vi "获取2号下位机4路温度值并显示和存进数据库.vi"() -> ()   [LabVIEW 2022 SP3]
uses:
  <vilib>/Instr/_visa.llb/VISA Configure Serial Port (Instr).vi
panel:
  out "所有测量记录":string[][](table)
  out "提取的第四路温度原始数据":string
  out "提取的第三路温度原始数据":string
  out "提取的第二路温度原始数据":string
  out "第一路温度值":dbl[](array[numeric])
  out "提取的第一路温度原始数据":string
  out "获取下位机返回的原始数据包":string
  in  "发送命令":string
  in  "波特率":u32=9600 caption="波特率(9600)"
  in  "选择串口":refnum<visa-resource-name>
  # "第二路温度值"
  # "第三路温度值"
  # "第四路温度值"
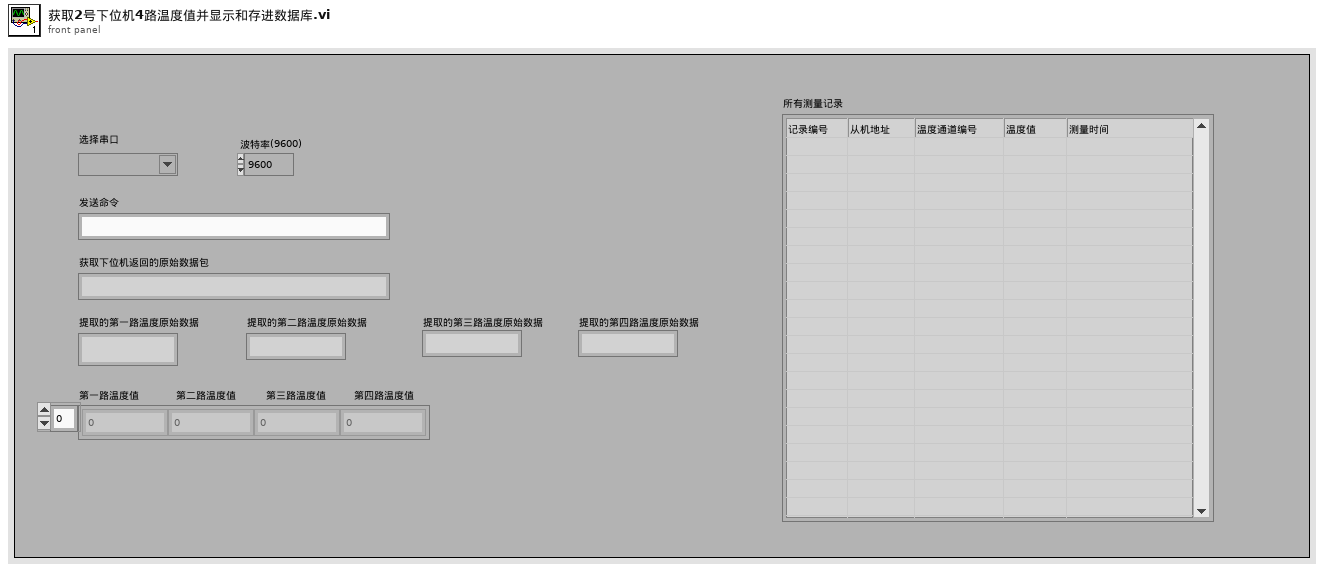
[diagram p1: front panel]
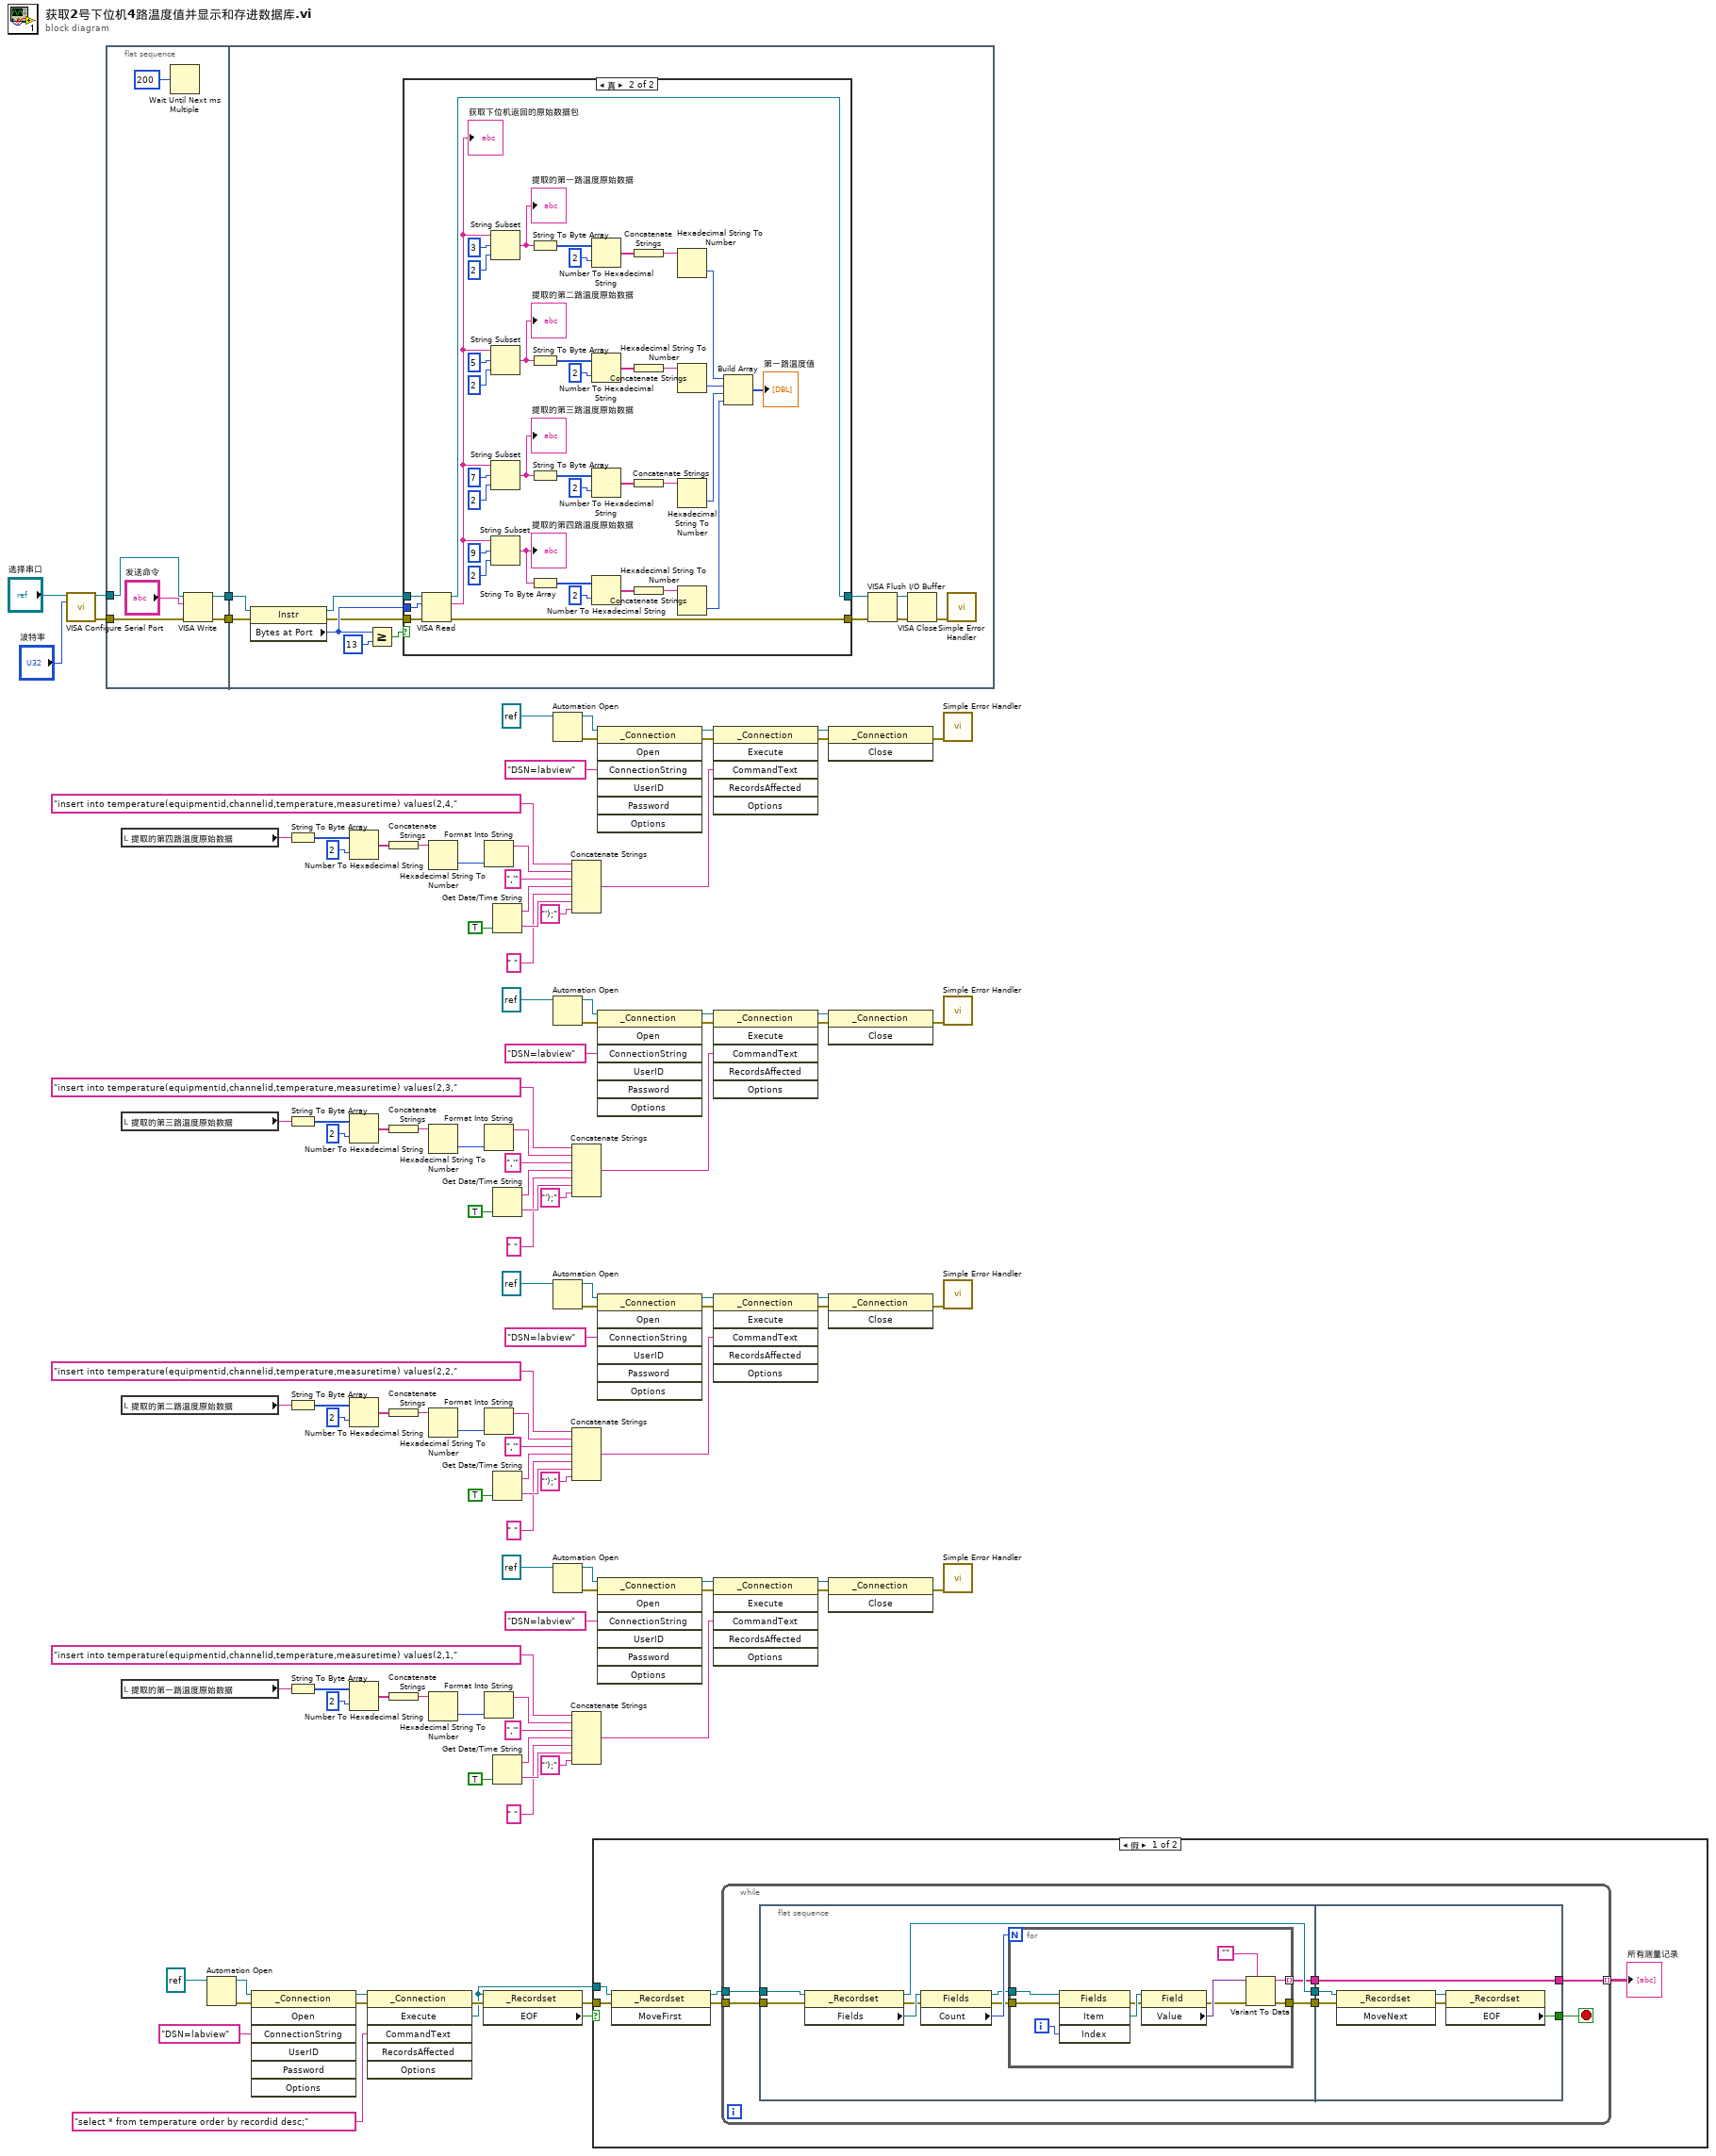
[diagram p0: block diagram]
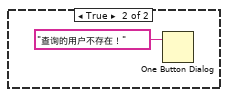
[diagram p2: hidden frame]
diagram:
  n1 = call-poly "VISA Configure Serial Port"("VISA resource name"="选择串口", "baud rate (9600)"="波特率") -> ("VISA resource name out"=w111:refnum<visa-resource-name>, "error out"=w110:errorcluster)  [unwired: 12 in]
  n2 = flat-sequence {
    tunnel: w111 -> [w118]
    tunnel: w110 -> [w117]
    tunnel: [w115] -> w109
    tunnel: [w114] -> w108
    tunnel: w109 -> [w131]
    tunnel: w108 -> [w130]
    frame #0 {
      n3 = Wait Until Next ms Multiple(millisecond multiple=u32 200 ("毫秒倍数")) -> ()  [unwired: 1 out]
      n4 = VISA Write(VISA resource name=w118, write buffer="发送命令", error in (no error)=w117) -> (VISA resource name out=w115:refnum<visa-resource-name>, error out=w114:errorcluster)  [unwired: 1 out]
    }
    frame #1 {
      n5 = property class="Instr"(reference=w131, error in=w130) -> (reference out=w127:refnum<visa-resource-name>, error out=w125:errorcluster, "Bytes at Port"=w126:u32)
      n6 = Greater Or Equal?(x=w126, y=u32 13) -> (x >= y?=w129:bool)
      n7 = case shown="真" w129 {
        tunnel: w127 -> [w133 w172]
        tunnel: w126 -> [_ w171]
        tunnel: w125 -> [w132 w170]
        tunnel: [w133 w162] -> w121
        tunnel: [w132 w161] -> w120
        frame False {
        }
        frame True {
          n8 = VISA Read(VISA resource name=w172, byte count=w171, error in (no error)=w170) -> (VISA resource name out=w162:refnum<visa-resource-name>, read buffer=w139:string, error out=w161:errorcluster)  [unwired: 1 out]
          "获取下位机返回的原始数据包" <- w139
          n9 = String Subset(string=w139, offset (0)=3 ("偏移量(0)"), length (rest)=2 ("长度（剩余）")) -> (substring=w167:string)
          "提取的第一路温度原始数据" <- w167
          n10 = String Subset(string=w139, offset (0)=5 ("偏移量(0)"), length (rest)=2 ("长度（剩余）")) -> (substring=w157:string)
          "提取的第二路温度原始数据" <- w157
          n11 = String Subset(string=w139, offset (0)=7 ("偏移量(0)"), length (rest)=2 ("长度（剩余）")) -> (substring=w150:string)
          "提取的第三路温度原始数据" <- w150
          n12 = String Subset(string=w139, offset (0)=9 ("偏移量(0)"), length (rest)=2 ("长度（剩余）")) -> (substring=w144:string)
          "提取的第四路温度原始数据" <- w144
          n13 = String To Byte Array(string=w167) -> (unsigned byte array=w166:u8[])
          n14 = String To Byte Array(string=w157) -> (unsigned byte array=w156:u8[])
          n15 = String To Byte Array(string=w150) -> (unsigned byte array=w149:u8[])
          n16 = String To Byte Array(string=w144) -> (unsigned byte array=w143:u8[])
          n17 = Number To Hexadecimal String(1:i16 2 ("宽度(-)"), 2:w166) -> (0:w164:string[])
          n18 = Number To Hexadecimal String(1:i16 2 ("宽度(-)"), 2:w156) -> (0:w154:string[])
          n19 = Number To Hexadecimal String(1:i16 2 ("宽度(-)"), 2:w149) -> (0:w147:string[])
          n20 = Number To Hexadecimal String(1:i16 2 ("宽度(-)"), 2:w143) -> (0:w141:string[])
          n21 = Concatenate Strings(w164) -> (w163:string)
          n22 = Concatenate Strings(w154) -> (w153:string)
          n23 = Concatenate Strings(w147) -> (w146:string)
          n24 = Concatenate Strings(w141) -> (w140:string)
          n25 = Hexadecimal String To Number(string=w163) -> (number=w134:u32)  [unwired: 2 in, 1 out]
          n26 = Hexadecimal String To Number(string=w153) -> (number=w137:u32)  [unwired: 2 in, 1 out]
          n27 = Hexadecimal String To Number(string=w146) -> (number=w136:u32)  [unwired: 2 in, 1 out]
          n28 = Hexadecimal String To Number(string=w140) -> (number=w135:u32)  [unwired: 2 in, 1 out]
          n29 = Build Array(w134, w137, w136, w135) -> (→"第一路温度值":u32[])
        }
      }
      n30 = VISA Flush I/O Buffer(VISA resource name=w121, error in (no error)=w120) -> (VISA resource name out=w122:refnum<visa-resource-name>, error out=w123:errorcluster)  [unwired: 1 in]
      n31 = VISA Close(VISA resource name=w122, error in (no error)=w123) -> (error out=w124:errorcluster)
      n32 = call <vilib>:"Simple Error Handler.vi"("error in (no error)"=w124) -> ()  [unwired: 4 in, 5 out]
    }
  }
  n33 = local read "提取的第四路温度原始数据"() -> (w1:string)
  n34 = local read "提取的第三路温度原始数据"() -> (w2:string)
  n35 = local read "提取的第二路温度原始数据"() -> (w49:string)
  n36 = local read "提取的第一路温度原始数据"() -> (w76:string)
  n37 = Automation Open(Automation Refnum=refnum<k7> refnum ("ADODB._Connection")) -> (Automation Refnum=w106:refnum<k7>, error out=w105:errorcluster)  [unwired: 3 in]
  n38 = invoke class="_Connection" method="Open"(reference=w106, error in=w105, "ConnectionString"="DSN=labview") -> (reference out=w103:refnum<k7>, error out=w102:errorcluster)  [unwired: 4 in, 5 out]
  n39 = String To Byte Array(string=w1) -> (unsigned byte array=w22:u8[])
  n40 = String To Byte Array(string=w2) -> (unsigned byte array=w45:u8[])
  n41 = String To Byte Array(string=w49) -> (unsigned byte array=w69:u8[])
  n42 = String To Byte Array(string=w76) -> (unsigned byte array=w93:u8[])
  n43 = Number To Hexadecimal String(1:i16 2 ("宽度(-)"), 2:w22) -> (0:w23:string[])
  n44 = Number To Hexadecimal String(1:i16 2 ("宽度(-)"), 2:w45) -> (0:w46:string[])
  n45 = Number To Hexadecimal String(1:i16 2 ("宽度(-)"), 2:w69) -> (0:w70:string[])
  n46 = Number To Hexadecimal String(1:i16 2 ("宽度(-)"), 2:w93) -> (0:w94:string[])
  n47 = invoke class="_Connection" method="Execute"(reference=w103, error in=w102, "CommandText"="select * from temperature order by recordid desc;") -> (error out=w100:errorcluster, "Execute"=w98:refnum<k7>)  [unwired: 3 in, 4 out]
  n48 = Concatenate Strings(w23) -> (w24:string)
  n49 = Concatenate Strings(w46) -> (w47:string)
  n50 = Concatenate Strings(w70) -> (w71:string)
  n51 = Concatenate Strings(w94) -> (w95:string)
  n52 = Hexadecimal String To Number(string=w24) -> (number=w25:u32)  [unwired: 2 in, 1 out]
  n53 = Hexadecimal String To Number(string=w47) -> (number=w48:u32)  [unwired: 2 in, 1 out]
  n54 = Hexadecimal String To Number(string=w71) -> (number=w72:u32)  [unwired: 2 in, 1 out]
  n55 = Hexadecimal String To Number(string=w95) -> (number=w96:u32)  [unwired: 2 in, 1 out]
  n56 = property class="_Recordset"(reference=w98, error in=w100) -> (error out=w97:errorcluster, "EOF"=w99:bool)  [unwired: 1 out]
  n57 = Format Into String(w25) -> (resulting string=w21:string)  [unwired: 3 in, 1 out]
  n58 = Format Into String(w48) -> (resulting string=w44:string)  [unwired: 3 in, 1 out]
  n59 = Format Into String(w72) -> (resulting string=w68:string)  [unwired: 3 in, 1 out]
  n60 = Format Into String(w96) -> (resulting string=w92:string)  [unwired: 3 in, 1 out]
  n61 = Get Date/Time String(want seconds? (F)=TRUE) -> (date string=w14:string, time string=w15:string)  [unwired: 2 in]
  n62 = Get Date/Time String(want seconds? (F)=TRUE) -> (date string=w37:string, time string=w38:string)  [unwired: 2 in]
  n63 = Get Date/Time String(want seconds? (F)=TRUE) -> (date string=w61:string, time string=w62:string)  [unwired: 2 in]
  n64 = Get Date/Time String(want seconds? (F)=TRUE) -> (date string=w85:string, time string=w86:string)  [unwired: 2 in]
  n65 = Automation Open(Automation Refnum=refnum<k7> refnum ("ADODB._Connection")) -> (Automation Refnum=w20:refnum<k7>, error out=w19:errorcluster)  [unwired: 3 in]
  n66 = Automation Open(Automation Refnum=refnum<k7> refnum ("ADODB._Connection")) -> (Automation Refnum=w43:refnum<k7>, error out=w42:errorcluster)  [unwired: 3 in]
  n67 = Automation Open(Automation Refnum=refnum<k7> refnum ("ADODB._Connection")) -> (Automation Refnum=w67:refnum<k7>, error out=w66:errorcluster)  [unwired: 3 in]
  n68 = Automation Open(Automation Refnum=refnum<k7> refnum ("ADODB._Connection")) -> (Automation Refnum=w91:refnum<k7>, error out=w90:errorcluster)  [unwired: 3 in]
  n69 = Concatenate Strings("insert into temperature(equipmentid,channelid,temperature,measuretime) values(2,4," ("CommandText"), w21, ",'" ("字符串"), w14, " " ("string"), w15, "');" ("string")) -> (w16:string)
  n70 = Concatenate Strings("insert into temperature(equipmentid,channelid,temperature,measuretime) values(2,3," ("CommandText"), w44, ",'" ("字符串"), w37, " " ("string"), w38, "');" ("string")) -> (w39:string)
  n71 = Concatenate Strings("insert into temperature(equipmentid,channelid,temperature,measuretime) values(2,2," ("CommandText"), w68, ",'" ("字符串"), w61, " " ("string"), w62, "');" ("string")) -> (w63:string)
  n72 = Concatenate Strings("insert into temperature(equipmentid,channelid,temperature,measuretime) values(2,1," ("CommandText"), w92, ",'" ("字符串"), w85, " " ("string"), w86, "');" ("string")) -> (w87:string)
  n73 = case shown="假" w99 {
    tunnel: w98 -> [w177 _]
    tunnel: w97 -> [w176 _]
    frame False {
      n74 = invoke class="_Recordset" method="MoveFirst"(reference=w177, error in=w176) -> (reference out=w174:refnum<k7>, error out=w175:errorcluster)  [unwired: 1 in, 1 out]
      n75 = while {
        tunnel: w175 -> [w182]
        tunnel: w174 -> [w181]
        tunnel: [w178] -> w173 mode=indexing
        stop <- w180 stop-if-true
        n76 = flat-sequence {
          tunnel: w181 -> [w194]
          tunnel: w182 -> [w193]
          tunnel: [w187] -> w184
          tunnel: [w186] -> w183
          tunnel: [w185] -> w179
          tunnel: w184 -> [w208]
          tunnel: w183 -> [w207]
          tunnel: [w206] -> w180
          tunnel: w179 -> [w205]
          tunnel: [w205] -> w178
          frame #0 {
            n77 = property class="_Recordset"(reference=w194, error in=w193) -> (reference out=w186:refnum<k7>, error out=w191:errorcluster, "Fields"=w192:refnum<k7>)
            n78 = property class="Fields"(reference=w192, error in=w191) -> (reference out=w189:refnum<k7>, error out=w188:errorcluster, "Count"=w190:i32)
            n79 = for {
              N: w190 -> [_]
              tunnel: w189 -> [w199]
              tunnel: w188 -> [w198]
              tunnel: [w196] -> w185 mode=indexing
              tunnel: [w195] -> w187
              i -> [w197]
              n80 = invoke class="Fields" method="Item"(reference=w199, error in=w198, "Index"=w197) -> (error out=w203:errorcluster, "Item"=w204:refnum<k7>)  [unwired: 1 in, 2 out]
              n81 = property class="Field"(reference=w204, error in=w203) -> (error out=w200:errorcluster, "Value"=w201:variant)  [unwired: 1 out]
              n82 = Variant To Data(error in=w200, type="", Variant=w201) -> (data=w196:string, error out=w195:errorcluster)
            }
          }
          frame #1 {
            n83 = invoke class="_Recordset" method="MoveNext"(reference=w207, error in=w208) -> (reference out=w210:refnum<k7>, error out=w209:errorcluster)  [unwired: 1 in, 1 out]
            n84 = property class="_Recordset"(reference=w210, error in=w209) -> ("EOF"=w206:bool)  [unwired: 2 out]
          }
        }
      }
      "所有测量记录" <- w173
    }
    frame True {
      n85 = One Button Dialog(message="查询的用户不存在！") -> ()  [unwired: 1 in, 1 out]
    }
  }
  n86 = invoke class="_Connection" method="Open"(reference=w20, error in=w19, "ConnectionString"="DSN=labview") -> (reference out=w18:refnum<k7>, error out=w17:errorcluster)  [unwired: 4 in, 5 out]
  n87 = invoke class="_Connection" method="Open"(reference=w43, error in=w42, "ConnectionString"="DSN=labview") -> (reference out=w41:refnum<k7>, error out=w40:errorcluster)  [unwired: 4 in, 5 out]
  n88 = invoke class="_Connection" method="Open"(reference=w67, error in=w66, "ConnectionString"="DSN=labview") -> (reference out=w65:refnum<k7>, error out=w64:errorcluster)  [unwired: 4 in, 5 out]
  n89 = invoke class="_Connection" method="Open"(reference=w91, error in=w90, "ConnectionString"="DSN=labview") -> (reference out=w89:refnum<k7>, error out=w88:errorcluster)  [unwired: 4 in, 5 out]
  n90 = invoke class="_Connection" method="Execute"(reference=w18, error in=w17, "CommandText"=w16) -> (reference out=w4:refnum<k7>, error out=w3:errorcluster)  [unwired: 3 in, 4 out]
  n91 = invoke class="_Connection" method="Execute"(reference=w41, error in=w40, "CommandText"=w39) -> (reference out=w27:refnum<k7>, error out=w26:errorcluster)  [unwired: 3 in, 4 out]
  n92 = invoke class="_Connection" method="Execute"(reference=w65, error in=w64, "CommandText"=w63) -> (reference out=w51:refnum<k7>, error out=w50:errorcluster)  [unwired: 3 in, 4 out]
  n93 = invoke class="_Connection" method="Execute"(reference=w89, error in=w88, "CommandText"=w87) -> (reference out=w74:refnum<k7>, error out=w73:errorcluster)  [unwired: 3 in, 4 out]
  n94 = invoke class="_Connection" method="Close"(reference=w4, error in=w3) -> (error out=w5:errorcluster)  [unwired: 1 in, 2 out]
  n95 = invoke class="_Connection" method="Close"(reference=w27, error in=w26) -> (error out=w28:errorcluster)  [unwired: 1 in, 2 out]
  n96 = invoke class="_Connection" method="Close"(reference=w51, error in=w50) -> (error out=w52:errorcluster)  [unwired: 1 in, 2 out]
  n97 = invoke class="_Connection" method="Close"(reference=w74, error in=w73) -> (error out=w75:errorcluster)  [unwired: 1 in, 2 out]
  n98 = call <vilib>:"Simple Error Handler.vi"("error in (no error)"=w5) -> ()  [unwired: 4 in, 5 out]
  n99 = call <vilib>:"Simple Error Handler.vi"("error in (no error)"=w28) -> ()  [unwired: 4 in, 5 out]
  n100 = call <vilib>:"Simple Error Handler.vi"("error in (no error)"=w52) -> ()  [unwired: 4 in, 5 out]
  n101 = call <vilib>:"Simple Error Handler.vi"("error in (no error)"=w75) -> ()  [unwired: 4 in, 5 out]
